vi "零点跨度数据组合 (子VI).vi"(8 "span value":string="0", 9 "standard value":string, 10 "check value":string, 11 "污染物编码":string) -> (3 "组合输出":string)   [LabVIEW 2016, in "数据传输系统-04.lvlib"]
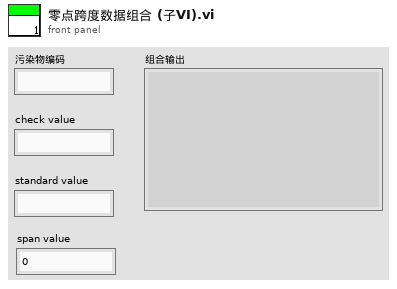
[diagram p1: front panel]
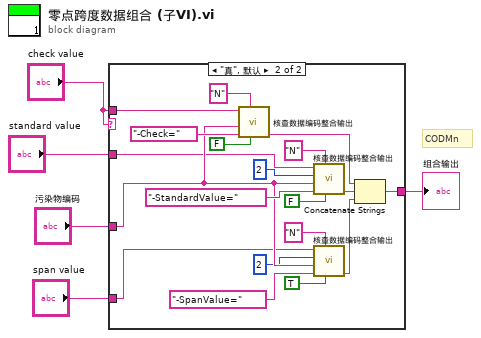
[diagram p0: block diagram]
diagram:
  # "CODMn"
  n1 = case shown="\"真\", 默认" "check value" {
    tunnel: "check value" -> [w6 w24]
    tunnel: [w6 w21] -> w2
    tunnel: "standard value" -> [_ w7]
    tunnel: "污染物编码" -> [_ w11]
    tunnel: "span value" -> [_ w8]
    frame "" {
    }
    frame "真", Default {
      n2 = call "核查数据编码整合输出.vi"("字段结束"=FALSE, "数据标识"="N" ("字符串"), "数据类型"="-Check=", "污染物编码"=w11, "数据值"=w24) -> ("编码输出"=w22:string)  [unwired: 6 in]
      n3 = call "核查数据编码整合输出.vi"("字段结束"=FALSE, "数据标识"="N" ("字符串"), "数据类型"="-StandardValue=", "污染物编码"=w11, "数据精度"=2, "数据值"=w7) -> ("编码输出"=w18:string)  [unwired: 5 in]
      n4 = call "核查数据编码整合输出.vi"("字段结束"=TRUE, "数据标识"="N" ("字符串"), "数据类型"="-SpanValue=", "污染物编码"=w11, "数据精度"=2, "数据值"=w8) -> ("编码输出"=w15:string)  [unwired: 5 in]
      n5 = Concatenate Strings(w22, w18, w15) -> (w21:string)
    }
  }
  "组合输出" <- w2
